vi "dfd_X to Power of 2.vi"(10 "x":dbl) -> (2 "2^n x":dbl, 5 "n":dbl, 7 "is 2^n?":bool)   [LabVIEW 2017, in "NI_DigFilterLicensed.lvlib"]
uses:
  <vilib>/addons/Digital Filter Design/NI_DigFilterLicensed.lvlib
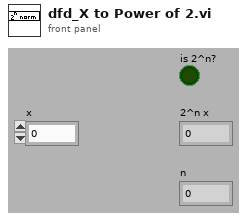
[diagram p1: front panel]
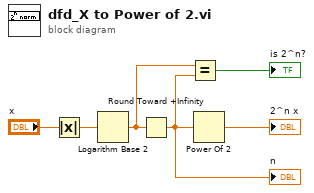
[diagram p0: block diagram]
diagram:
  n1 = Absolute Value(x="x") -> (abs(x)=w1:dbl)
  n2 = Logarithm Base 2(1:w1) -> (0:w4:dbl)
  n3 = Round Toward +Infinity(x=w4) -> (ceil(x): smallest int >= x=w3:dbl)
  "n" <- w3
  n4 = Equal?(x=w4, y=w3) -> (x = y?=→"is 2^n?":bool)
  n5 = Power Of 2(x=w3) -> (2^x=→"2^n x":dbl)
